vi "Read Measure All Devices--SubVI.vi"(8 "error in (no error)":errorcluster, 11 "Flexi-Flow in":T1 {"Control State"."Control Mode" items=["Bus/RS232"=0, "FLOW-BUS slave"=2, "Valve close"=3, "Controller idle"=4, "Setpoint 100%"=7, "Valve fully open"=8, "Calibration mode"=9, "Setpoint 0%"=12, "RS232"=18, "Valve steering"=20, "Valve safe state"=22]}) -> (0 "error out":errorcluster, 1 "Value":sgl, 2 "map out":map{string, dbl}(c390), 3 "Flexi-Flow out":T1 {"Control State"."Control Mode" items=["Bus/RS232"=0, "FLOW-BUS slave"=2, "Valve close"=3, "Controller idle"=4, "Setpoint 100%"=7, "Valve fully open"=8, "Calibration mode"=9, "Setpoint 0%"=12, "RS232"=18, "Valve steering"=20, "Valve safe state"=22]})   [LabVIEW 2024, in "FlexiFlowInterface.lvlib"]
uses:
  FlexiFlowInterface.lvlib
  Modbus Flexi-Flow State--cluster.ctl
  <vilib>/Plasmionique/MB Master/MB_Master_TCP/MB_Master_TCP.lvclass
  Device Type--enum.ctl
  Modbus Flexi-Flow Controls--cluster.ctl
  Modbus Flexi-Flow API/Control Mode--enum.ctl
  Modbus Flexi-Flow API/Control Function Values--enum.ctl
  Modbus Flexi-Flow Measure State--cluster.ctl
  Modbus Flexi-Flow API/Bronkhorst Flexi-Flow ModbusTCP API.lvlib
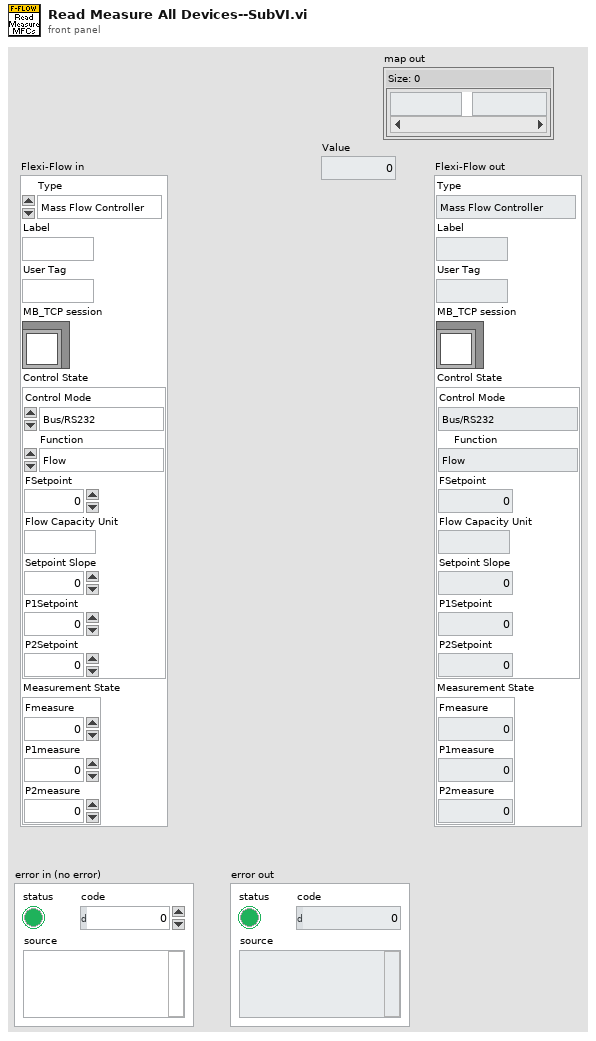
[diagram p1: front panel]
types:
  T1 = typedef "FlexiFlowInterface.lvlib/Modbus Flexi-Flow State--cluster.ctl" = cluster{"Type":T2, "Label":string, "User Tag":string, "MB_TCP session":refnum<class "MB_Master_TCP.lvclass">, "Control State":T3, "Measurement State":T6}
  T2 = typedef "FlexiFlowInterface.lvlib/Device Type--enum.ctl" = enum16{"Mass Flow Controller", "Mass Flow Meter"}
  T3 = typedef "FlexiFlowInterface.lvlib/Modbus Flexi-Flow Controls--cluster.ctl" = cluster{"Control Mode":T4, "Function":T5, "FSetpoint":sgl, "Flow Capacity Unit":string, "Setpoint Slope":u16, "P1Setpoint":sgl, "P2Setpoint":sgl}
  T4 = typedef "Bronkhorst Flexi-Flow ModbusTCP API.lvlib/Control Mode--enum.ctl" = u16
  T5 = typedef "Bronkhorst Flexi-Flow ModbusTCP API.lvlib/Control Function Values--enum.ctl" = enum16{"Flow", "Upstream pressure", "Downstream pressure", "Flow with upstream pressure limit", "Flow with downstream pressure limit", "Upstream pressure with flow limit", "Downstream pressure with flow limit"}
  T6 = typedef "FlexiFlowInterface.lvlib/Modbus Flexi-Flow Measure State--cluster.ctl" = cluster{"Fmeasure":dbl, "P1measure":sgl, "P2measure":sgl}
  T7 = typedef "Bronkhorst Flexi-Flow ModbusTCP API.lvlib/Fmeasure (F,P1,P2)--cluster.ctl" = cluster{"Fmeasure (F)":sgl, "Fmeasure (P1)":sgl, "Fmeasure (P2)":sgl}
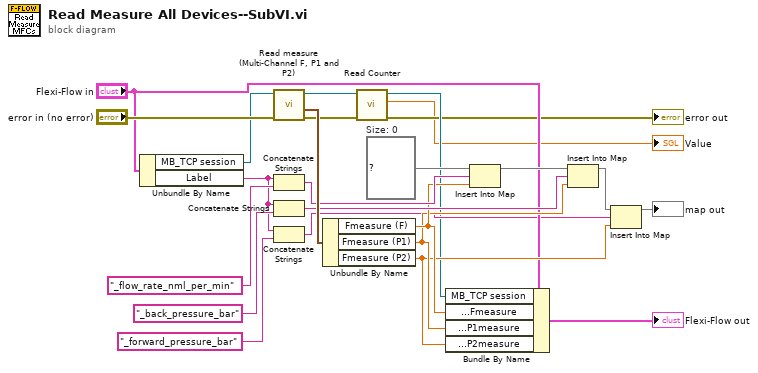
[diagram p0: block diagram]
diagram:
  w20 = map{string, dbl} {}  # Size: 0
  n1 = Unbundle By Name("Flexi-Flow in") -> ("MB_TCP session"=w21:refnum<class "MB_Master_TCP.lvclass">, "Label"=w8:string)
  n2 = call "Read measure (Multi-Channel F, P1 and P2).vi"("error in"="error in (no error)", "MB_TCP session in"=w21) -> ("error out"=w3:errorcluster, "Fmeasure (F, P1, P2)"=w23:T7, "MB session out"=w5:refnum<class "MB_Master_TCP.lvclass">)  [unwired: 7 in]
  n3 = Concatenate Strings(w8, "_flow_rate_nml_per_min" ("string")) -> (w18:string)
  n4 = Concatenate Strings(w8, "_back_pressure_bar" ("string")) -> (w15:string)
  n5 = Concatenate Strings(w8, "_forward_pressure_bar" ("key")) -> (w6:string)
  n6 = Unbundle By Name(w23) -> ("Fmeasure (F)"=w13:sgl, "Fmeasure (P1)"=w12:sgl, "Fmeasure (P2)"=w11:sgl)
  n7 = call "Read Counter.vi"("error in"=w3, "MB_TCP session in"=w5) -> ("error out"=→"error out":errorcluster, "Value"=→"Value":sgl, "MB session out"=w4:refnum<class "MB_Master_TCP.lvclass">)  [unwired: 7 in]
  n8 = Bundle By Name(cluster="Flexi-Flow in", "MB_TCP session"=w4, "Measurement State.Fmeasure"=w13, "Measurement State.P1measure"=w12, "Measurement State.P2measure"=w11) -> (→"Flexi-Flow out":T1)
  n9 = Insert Into Map(map in=w20, key=w18, value=w13) -> (map out=w17:map{string, dbl})  [unwired: 2 out]
  n10 = Insert Into Map(map in=w17, key=w15, value=w12) -> (map out=w14:map{string, dbl})  [unwired: 2 out]
  n11 = Insert Into Map(map in=w14, key=w6, value=w11) -> (map out=→"map out":map{string, dbl})  [unwired: 2 out]
